vi "4-3.vi"(1 "输入":dbl) -> (0 "输出":dbl)   [LabVIEW 2017]
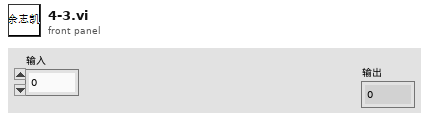
[diagram p1: front panel]
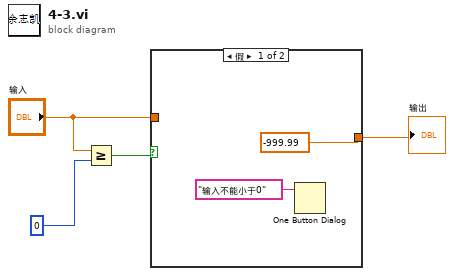
[diagram p0: block diagram]
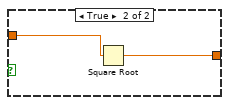
[diagram p2: hidden frame]
diagram:
  n1 = Greater Or Equal?(x="输入", y=0) -> (x >= y?=w1:bool)
  n2 = case shown="假" w1 {
    tunnel: "输入" -> [_ w8]
    tunnel: [-999.99 w7] -> w2
    frame False {
      n3 = One Button Dialog(message="输入不能小于0") -> ()  [unwired: 1 in, 1 out]
    }
    frame True {
      n4 = Square Root(x=w8) -> (sqrt(x)=w7:dbl)
    }
  }
  "输出" <- w2
